vi "TwoBendingAmpMax.vi"(4 "phi 2":dbl, 6 "phi 1":dbl, 7 "2nd Mode Bending Options":u16(ring) items=["Specifiy Tail Amplitude & 1st Mode", "Specifiy Tail Amplitude & 2nd Mode"], 8 "Amp2 In":dbl, 9 "Amp1 In":dbl, 10 "Tail Amplitude":dbl, 11 "nL":dbl) -> (0 "Amp2 Out":dbl, 3 "Amp1 Out":dbl)   [LabVIEW 2017]
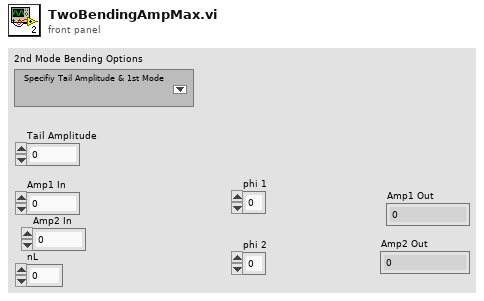
[diagram p1: front panel]
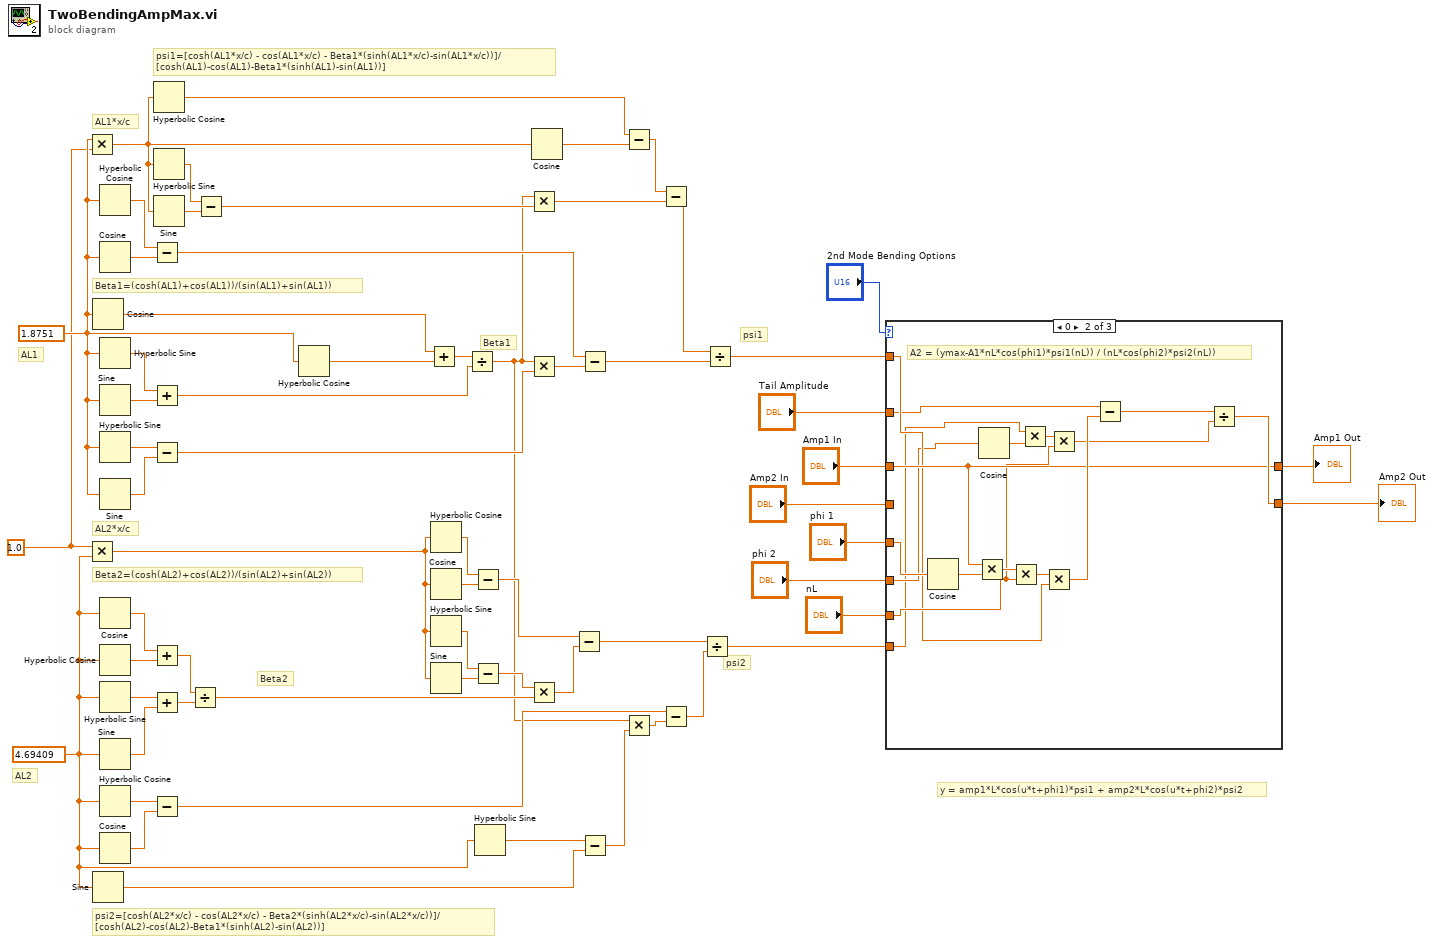
[diagram p0: block diagram]
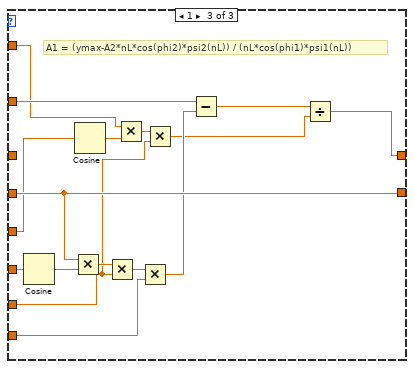
[diagram p3: hidden frame]
diagram:
  w12 = 1.0
  w23 = 4.69409
  w41 = 1.8751
  # "y = amp1*L*cos(u*t+phi1)*psi1 + amp2*L*cos(u*t+phi2)*psi2"
  # "psi1"
  # "psi2"
  # "AL2*x/c"
  # "AL1*x/c"
  # "psi2=[cosh(AL2*x/c) - cos(AL2*x/c) - Beta2*(sinh(AL2*x/c)-sin(AL2*x/c))]/\n[cosh(AL2)-cos(AL2)-Beta1*(sinh(AL2)-sin(AL2))]"
  # "psi1=[cosh(AL1*x/c) - cos(AL1*x/c) - Beta1*(sinh(AL1*x/c)-sin(AL1*x/c))]/\n[cosh(AL1)-cos(AL1)-Beta1*(sinh(AL1)-sin(AL1))]"
  # "Beta2=(cosh(AL2)+cos(AL2))/(sin(AL2)+sin(AL2))"
  # "Beta1=(cosh(AL1)+cos(AL1))/(sin(AL1)+sin(AL1))"
  # "Beta2"
  # "Beta1"
  # "AL2"
  # "AL1"
  n1 = Multiply(x=w41, y=w12) -> (x*y=w50:dbl)
  n2 = Multiply(x=w12, y=w23) -> (x*y=w24:dbl)
  n3 = Cosine(x=w41) -> (cos(x)=w61:dbl)
  n4 = Sine(x=w23) -> (sin(x)=w25:dbl)
  n5 = Hyperbolic Cosine(1:w41) -> (0:w40:dbl)
  n6 = Cosine(x=w41) -> (cos(x)=w39:dbl)
  n7 = Hyperbolic Sine(1:w41) -> (0:w60:dbl)
  n8 = Sine(x=w41) -> (sin(x)=w59:dbl)
  n9 = Hyperbolic Sine(1:w41) -> (0:w38:dbl)
  n10 = Sine(x=w41) -> (sin(x)=w37:dbl)
  n11 = Cosine(x=w23) -> (cos(x)=w57:dbl)
  n12 = Hyperbolic Cosine(1:w23) -> (0:w58:dbl)
  n13 = Hyperbolic Sine(1:w23) -> (0:w56:dbl)
  n14 = Sine(x=w23) -> (sin(x)=w55:dbl)
  n15 = Hyperbolic Cosine(1:w23) -> (0:w28:dbl)
  n16 = Cosine(x=w23) -> (cos(x)=w27:dbl)
  n17 = Subtract(x=w40, y=w39) -> (x-y=w34:dbl)
  n18 = Add(x=w60, y=w59) -> (x+y=w53:dbl)
  n19 = Subtract(x=w38, y=w37) -> (x-y=w36:dbl)
  n20 = Add(x=w57, y=w58) -> (x+y=w52:dbl)
  n21 = Add(x=w56, y=w55) -> (x+y=w51:dbl)
  n22 = Subtract(x=w28, y=w27) -> (x-y=w16:dbl)
  n23 = Hyperbolic Cosine(1:w50) -> (0:w46:dbl)
  n24 = Hyperbolic Sine(1:w50) -> (0:w49:dbl)
  n25 = Sine(x=w50) -> (sin(x)=w48:dbl)
  n26 = Divide(x=w52, y=w51) -> (x/y=w22:dbl)
  n27 = Subtract(x=w49, y=w48) -> (x-y=w47:dbl)
  n28 = Hyperbolic Cosine(1:w41) -> (0:w62:dbl)
  n29 = Add(x=w61, y=w62) -> (x+y=w54:dbl)
  n30 = Hyperbolic Cosine(1:w24) -> (0:w30:dbl)
  n31 = Cosine(x=w24) -> (cos(x)=w29:dbl)
  n32 = Hyperbolic Sine(1:w24) -> (0:w32:dbl)
  n33 = Sine(x=w24) -> (sin(x)=w31:dbl)
  n34 = Divide(x=w54, y=w53) -> (x/y=w13:dbl)
  n35 = Subtract(x=w30, y=w29) -> (x-y=w19:dbl)
  n36 = Subtract(x=w32, y=w31) -> (x-y=w21:dbl)
  n37 = Hyperbolic Sine(1:w23) -> (0:w26:dbl)
  n38 = Multiply(x=w13, y=w47) -> (x*y=w43:dbl)
  n39 = Multiply(x=w13, y=w36) -> (x*y=w35:dbl)
  n40 = Multiply(x=w21, y=w22) -> (x*y=w18:dbl)
  n41 = Cosine(x=w50) -> (cos(x)=w45:dbl)
  n42 = Subtract(x=w19, y=w18) -> (x-y=w17:dbl)
  n43 = Subtract(x=w34, y=w35) -> (x-y=w33:dbl)
  n44 = Subtract(x=w26, y=w25) -> (x-y=w15:dbl)
  n45 = Subtract(x=w46, y=w45) -> (x-y=w44:dbl)
  n46 = Multiply(x=w13, y=w15) -> (x*y=w14:dbl)
  n47 = Subtract(x=w44, y=w43) -> (x-y=w42:dbl)
  n48 = Subtract(x=w16, y=w14) -> (x-y=w20:dbl)
  n49 = Divide(x=w17, y=w20) -> (x/y=w2:dbl)
  n50 = Divide(x=w42, y=w33) -> (x/y=w3:dbl)
  n51 = case shown="0" "2nd Mode Bending Options" {
    tunnel: [w64 w71 w81] -> w8
    tunnel: "Amp1 In" -> [w64 w71 _]
    tunnel: [w63 w72 w92] -> w7
    tunnel: "Amp2 In" -> [w63 _ w92]
    tunnel: "Tail Amplitude" -> [_ w65 w96]
    tunnel: "phi 1" -> [_ w70 w87]
    tunnel: "phi 2" -> [_ w67 w94]
    tunnel: w3 -> [_ w68 w85]
    tunnel: w2 -> [_ w66 w89]
    tunnel: "nL" -> [_ w69 w83]
    frame Default {
    }
    frame 0 {
      # "A2 = (ymax-A1*nL*cos(phi1)*psi1(nL)) / (nL*cos(phi2)*psi2(nL))"
      n52 = Cosine(x=w70) -> (cos(x)=w79:dbl)
      n53 = Multiply(x=w71, y=w79) -> (x*y=w78:dbl)
      n54 = Cosine(x=w67) -> (cos(x)=w75:dbl)
      n55 = Multiply(x=w78, y=w69) -> (x*y=w77:dbl)
      n56 = Multiply(x=w66, y=w75) -> (x*y=w74:dbl)
      n57 = Multiply(x=w77, y=w68) -> (x*y=w76:dbl)
      n58 = Multiply(x=w74, y=w69) -> (x*y=w73:dbl)
      n59 = Subtract(x=w65, y=w76) -> (x-y=w80:dbl)
      n60 = Divide(x=w80, y=w73) -> (x/y=w72:dbl)
    }
    frame 1 {
      # "A1 = (ymax-A2*nL*cos(phi2)*psi2(nL)) / (nL*cos(phi1)*psi1(nL))"
      n61 = Cosine(x=w94) -> (cos(x)=w93:dbl)
      n62 = Multiply(x=w92, y=w93) -> (x*y=w91:dbl)
      n63 = Cosine(x=w87) -> (cos(x)=w86:dbl)
      n64 = Multiply(x=w91, y=w83) -> (x*y=w90:dbl)
      n65 = Multiply(x=w85, y=w86) -> (x*y=w84:dbl)
      n66 = Multiply(x=w90, y=w89) -> (x*y=w88:dbl)
      n67 = Multiply(x=w84, y=w83) -> (x*y=w82:dbl)
      n68 = Subtract(x=w96, y=w88) -> (x-y=w95:dbl)
      n69 = Divide(x=w95, y=w82) -> (x/y=w81:dbl)
    }
  }
  "Amp1 Out" <- w8
  "Amp2 Out" <- w7
